vi "Utility - Configuration File Generator.vi"() -> ()   [LabVIEW 2015]
uses:
  <vilib>/LabVIEW Targets/FPGA/cRIO/shared/nicrio_ModuleControls/nicrio_cRIO-9234_DataRatesRing2.ctl
  controls/TDMS Properties.ctl
  controls/Acquisition and Logging Configuration.ctl
  <vilib>/Utility/xml.llb/Write to XML File(string).vi
panel:
  in  "TDMS Properties":T1[](array[typedef])=[{"Name"="Enterprise", "Value"="[CompanyName]"}, {"Name"="Author", "Value"="[DeveloperName]"}, {"Name"="Operator", "Value"="[OperatorName]"}, {"Name"="TestSystem", "Value"="[SystemName]"}, {"Name"="Site", "Value"="[Location]"}, {"Name"="Line", "Value"="[Line]"}, {"Name"="Machine", "Value"="[MachineName]"}, {"Name"="Description", "Value"="[Description]"}]
  in  "Trigger - Time (Minute)":i32=30
  in  "Trigger - Channel":i32
  in  "Trigger - RMS Value":dbl=1.8
  in  "Channel Names":string[](array[string])=["Mod1/ai0", "Mod1/ai1", "Mod1/ai2", "Mod1/ai3", "Mod2/ai0", "Mod2/ai1", "Mod2/ai2", "Mod2/ai3", "Mod3/ai0", "Mod3/ai1", "Mod3/ai2", "Mod3/ai3", "Mod4/ai0", "Mod4/ai1", "Mod4/ai2", "Mod4/ai3", "Mod5/ai0", "Mod5/ai1", "Mod5/ai2", "Mod5/ai3", "Mod6/ai0", "Mod6/ai1", "Mod6/ai2", "Mod6/ai3"]
  in  "Channel Scale Array":fxp<+,24,12>[](array[numeric])=[1.0, 1.0, 1.0, 2.0, 1.0, 1.0, 1.0, 2.0, 1.0, 1.0, 1.0, 2.0, 1.0, 1.0, 1.0, 2.0, 1.0, 1.0, 1.0, 2.0, 1.0, 1.0, 1.0, 2.0]
  in  "Number of Channels":i32=24
  in  "Data File Name":string="cRIO_Data"
  in  "Number of Reads to Save":i32=20
  in  "Samples per Read":i32=12800
  in  "Data Rate":T2=1 items=["51.200 kS/s (NI 9234)"=1, "25.600 kS/s (NI 9234)"=2, "17.067 kS/s (NI 9234)"=3, "12.800 kS/s (NI 9234)"=4, "10.240 kS/s (NI 9234)"=5, "8.533 kS/s (NI 9234)"=6, "7.314 kS/s (NI 9234)"=7, "6.400 kS/s (NI 9234)"=8, "5.689 kS/s (NI 9234)"=9, "5.120 kS/s (NI 9234)"=10, "4.654 kS/s (NI 9234)"=11, "4.267 kS/s (NI 9234)"=12, "3.938 kS/s (NI 9234)"=13, "3.657 kS/s (NI 9234)"=14, "3.413 kS/s (NI 9234)"=15, "3.200 kS/s (NI 9234)"=16, "3.012 kS/s (NI 9234)"=17, "2.845 kS/s (NI 9234)"=18, "2.695 kS/s (NI 9234)"=19, "2.560 kS/s (NI 9234)"=20, "2.438 kS/s (NI 9234)"=21, "2.328 kS/s (NI 9234)"=22, "2.226 kS/s (NI 9234)"=23, "2.133 kS/s (NI 9234)"=24, "2.048 kS/s (NI 9234)"=25, "1.969 kS/s (NI 9234)"=26, "1.896 kS/s (NI 9234)"=27, "1.829 kS/s (NI 9234)"=28, "1.765 kS/s (NI 9234)"=29, "1.707 kS/s (NI 9234)"=30, "1.652 kS/s (NI 9234)"=31]
  # "Instructions: Populate the controls below with desired values, then run the VI to generate a 'Config.xml' file in the root folder of your project.  \n\nNote:  Once you have generated the Config.xml file, you will need to copy it to the root folder of your RT Target."
  # "Acquisition"
  # "Channels"
  # "Logging"
  # "Trigger"
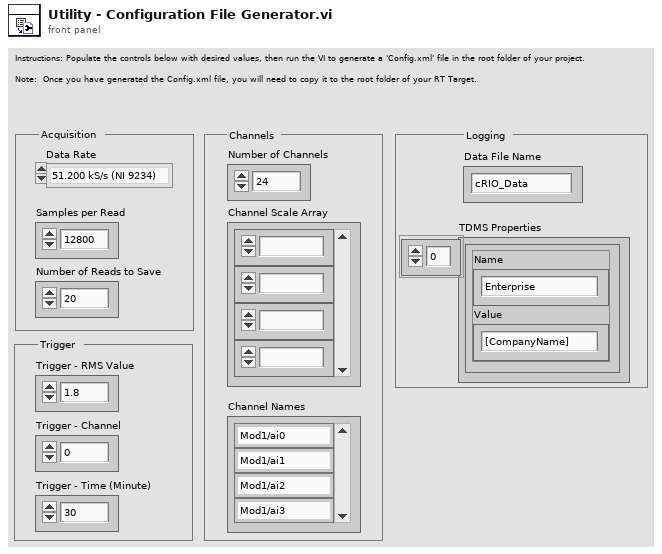
[diagram p1: front panel]
types:
  T1 = typedef "TDMS Properties.ctl" = cluster{"Name":string, "Value":string}
  T2 = typedef "nicrio_cRIO-9234_DataRatesRing2.ctl" = u8
  T3 = typedef "Acquisition and Logging Configuration.ctl" = cluster{"Data Rate":T2, "Samples per Read":i32, "Number of Reads to Save":i32, "Data File Name":string, "TDMS Properties":T1[], "Number of Channels":i32, "Channel Scale Array":fxp<+,24,12>[], "Channel Names":string[], "Trigger - RMS Value":dbl, "Trigger - Channel":i32, "Trigger - Time (Minute)":i32}
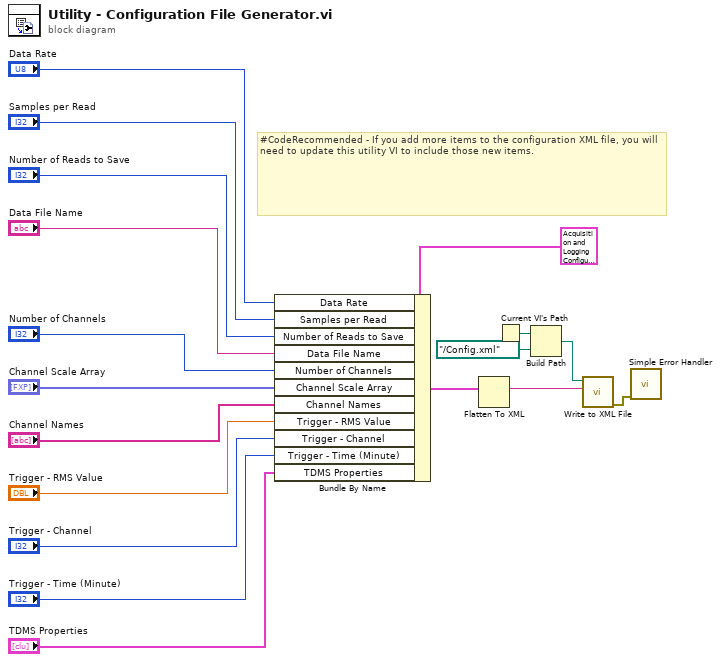
[diagram p0: block diagram]
diagram:
  # "#CodeRecommended - If you add more items to the configuration XML file, you will need to update this utility VI to include those new items."
  n1 = Bundle By Name(cluster=T3 {"Data Rate"=1, "Samples per Read"=0, "Number of Reads to Save"=0, "Data File Name"="", "TDMS Properties"=[], "Number of Channels"=0, "Channel Scale Array"=[0.0, 0.0, 0.0, 0.0, 1.0, 1.0, 1.0, 1.0, 1.0, 1.0, 1.0, 1.0, 1.0, 1.0, 1.0, 1.0, 1.0, 1.0, 1.0, 1.0, 1.0, 1.0, 1.0, 1.0], "Channel Names"=[], "Trigger - RMS Value"=0.0, "Trigger - Channel"=0, "Trigger - Time (Minute)"=0} ("Acquisition and Logging Configuration"), "Data Rate"="Data Rate", "Samples per Read"="Samples per Read", "Number of Reads to Save"="Number of Reads to Save", "Data File Name"="Data File Name", "Number of Channels"="Number of Channels", "Channel Scale Array"="Channel Scale Array", "Channel Names"="Channel Names", "Trigger - RMS Value"="Trigger - RMS Value", "Trigger - Channel"="Trigger - Channel", "Trigger - Time (Minute)"="Trigger - Time (Minute)", "TDMS Properties"="TDMS Properties") -> (w1:T3)
  n2 = Flatten To XML(anything=w1) -> (xml string=w17:string)
  n3 = Current VI's Path() -> (path=w16:path)
  n4 = Build Path(base path=w16, name or relative path=path "../Config.xml") -> (appended path=w14:path)
  n5 = call-poly <vilib>:"Write to XML File.vi"("XML Input"=w17, "XML File Path"=w14) -> ("error out"=w13:errorcluster)  [unwired: 7 in, 2 out]
  n6 = call <vilib>:"Simple Error Handler.vi"("error in (no error)"=w13) -> ()  [unwired: 4 in, 5 out]
